vi "CONSTANT - lvBuild Version.vi"() -> (2 "Version":string="v1.0.0")   [LabVIEW 2014, in "G CLI LvBuild.lvlib"]
uses:
  G CLI LvBuild.lvlib
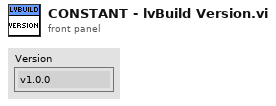
[diagram p1: front panel]
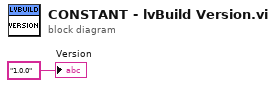
[diagram p0: block diagram]
diagram:
  "Version" <- "1.0.0"
